vi "DEMO - Command Listener.vi"() -> ()   [LabVIEW 2012]
uses:
  Alpha Command/STYP - Command Data Element.ctl
  <vilib>/Analysis/3filter.llb/Butterworth Filter (DBL).vi
  _REx/Components/Local Listener Session/Local Listener Session.lvclass
  Alpha Command/Alpha Cmd.lvclass
  Beta Command/Beta Cmd.lvclass
  <vilib>/Analysis/NI_AALBase.lvlib
panel:
  out "reversed":T1
  out "Waveform Graph":dbl[][](graph)
  out "error out":errorcluster
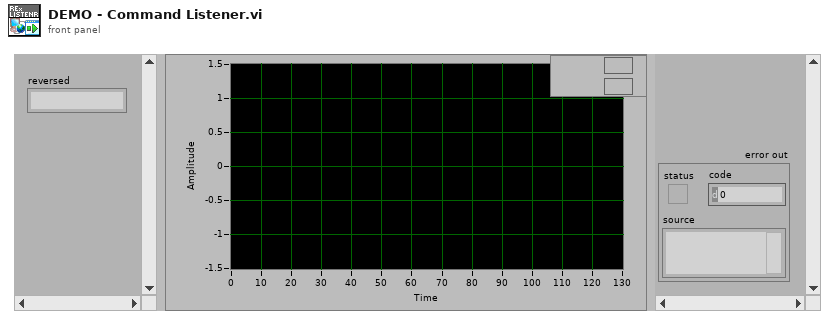
[diagram p1: front panel]
types:
  T1 = typedef "Alpha Cmd.lvclass/STYP - Command Data Element.ctl" = string
  T2 = typedef "REx.lvlib/Local Listener Session.lvclass/Session Handle.ctl" = refnum<data-value>
  T3 = typedef "Beta Cmd.lvclass/STYP - Command Data Element.ctl" = dbl[]
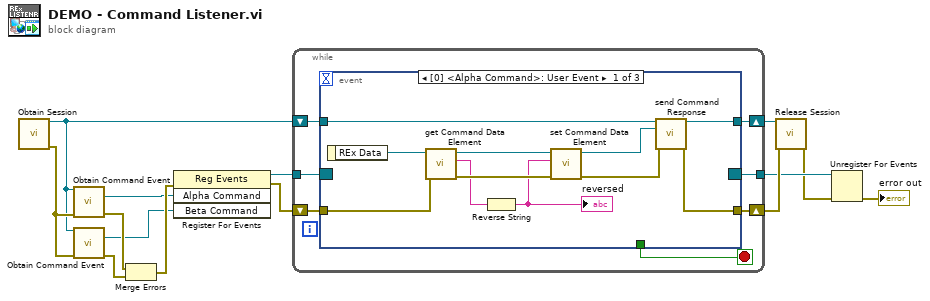
[diagram p0: block diagram]
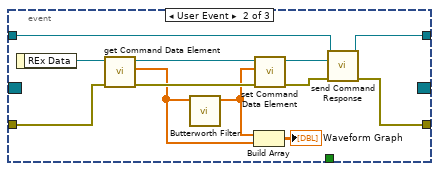
[diagram p2: hidden frame]
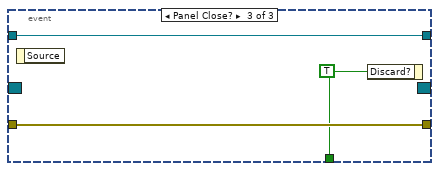
[diagram p3: hidden frame]
diagram:
  n1 = call "Obtain Session.vi"() -> ("Listener Session Handle"=w6:T2, "error out"=w14:errorcluster)  [unwired: 12 in, 2 out]
  n2 = call "Obtain Command Event.vi"("Local Listener Session"=w6, "error in (no error)"=w14) -> ("Alpha Command"=w3:refnum<user-event>, "error out"=w9:errorcluster)  [unwired: 12 in]
  n3 = call "Obtain Command Event.vi"("Local Listener Session"=w6, "error in (no error)"=w14) -> ("Beta Command"=w2:refnum<user-event>, "error out"=w8:errorcluster)  [unwired: 12 in]
  n4 = Merge Errors(w9, w8) -> (w7:errorcluster)
  n5 = register-events(error in=w7, w3, w2) -> (reference out=w11:refnum<event-registration>, error out=w13:errorcluster)  [unwired: 1 in]
  n6 = while {
    tunnel: w11 -> [w16]
    shift-right: [w20] -> w12
    shift-left: w6 -> [w21]
    shift-right: [w18] -> w10
    shift-left: w13 -> [w17]
    tunnel: [w15] -> w5
    stop <- w19 stop-if-true
    n7 = event shown="[0] <Alpha Command>: User Event" {
      selector: w16 -> [_ _ _]
      dyn-events: [_ _ _] -> w15
      timeout: _ -> [_ _ _]
      tunnel: w21 -> [w32 w34 w47]
      tunnel: [w31 w33 w47] -> w20
      tunnel: [_ _ w45] -> w19
      tunnel: [w30 w35 w46] -> w18
      tunnel: w17 -> [w28 w41 w46]
      event User Event {
        n8 = event-data() -> ("REx Data"=w29:refnum<class "Alpha Cmd.lvclass">)  [unwired: 1 in]
        n9 = call "get Command Data Element.vi"("error in (no error)"=w28, "REx - CMD_TEMPLATE in"=w29) -> ("error out"=w26:errorcluster, "Command Data Element"=w23:T1, "REx - CMD_TEMPLATE out"=w27:refnum<class "Alpha Cmd.lvclass">)  [unwired: 7 in]
        n10 = Reverse String(1:w23) -> (0:w22:T1)
        "reversed" <- w22
        n11 = call "set Command Data Element.vi"("error in (no error)"=w26, "Command Data Element"=w22, "REx - CMD_TEMPLATE in"=w27) -> ("error out"=w24:errorcluster, "REx - CMD_TEMPLATE out"=w25:refnum<class "Alpha Cmd.lvclass">)  [unwired: 7 in]
        n12 = call "send Command Response.vi"("Listener Handle in"=w32, "REx Command"=w25, "error in (no error)"=w24) -> ("Listener Handle out"=w31:T2, "error out"=w30:errorcluster)  [unwired: 11 in]
      }
      event User Event {
        n13 = event-data() -> ("REx Data"=w44:refnum<class "Beta Cmd.lvclass">)  [unwired: 1 in]
        n14 = call "get Command Data Element.vi"("error in (no error)"=w41, "REx - CMD_TEMPLATE in"=w44) -> ("error out"=w40:errorcluster, "Command Data Element"=w39:T3, "REx - CMD_TEMPLATE out"=w43:refnum<class "Beta Cmd.lvclass">)  [unwired: 7 in]
        n15 = call-poly <vilib>:"Butterworth Filter.vi"("X"=w39) -> ("Filtered X"=w38:dbl[])  [unwired: 7 in, 1 out]
        n16 = Build Array(w38, w39) -> (→"Waveform Graph":dbl[][])
        n17 = call "set Command Data Element.vi"("error in (no error)"=w40, "Command Data Element"=w38, "REx - CMD_TEMPLATE in"=w43) -> ("error out"=w36:errorcluster, "REx - CMD_TEMPLATE out"=w42:refnum<class "Beta Cmd.lvclass">)  [unwired: 7 in]
        n18 = call "send Command Response.vi"("Listener Handle in"=w34, "REx Command"=w42, "error in (no error)"=w36) -> ("Listener Handle out"=w33:T2, "error out"=w35:errorcluster)  [unwired: 11 in]
      }
      event Panel Close? {
        w45 = TRUE
        n19 = event-data() -> ()  [unwired: 1 in, 1 out]
        n20 = event-data("Discard?"=w45) -> ()  [unwired: 1 in, 1 out]
      }
    }
  }
  n21 = call "Release Session.vi"("Session Handle"=w12, "error in (no error)"=w10) -> ("error out"=w4:errorcluster)  [unwired: 13 in]
  n22 = Unregister For Events(event registration refnum=w5, error in=w4) -> (error out=→"error out":errorcluster)
